vi "Crio9067_4chan.vi"() -> ()   [LabVIEW 2014]
uses:
  <vilib>/rvi/eio/common/nirviEmuClasses.ctl
  <vilib>/rvi/Emulation/niFpgaGetClockAttributes.vi
  <vilib>/rvi/Emulation/niFpgaSctlEmulationGetInTimedLoop.vi
  <vilib>/rvi/Emulation/niFpgaEmulationReportErrorSimple.vi
  <vilib>/rvi/Emulation/niFpgaProcessEmulError.vi
  <vilib>/rvi/eio/common/nirviEmuTemplateMethod_errors.vi
  <vilib>/rvi/Emulation/niFpgaCriticalErrorInLSC.vi
  <vilib>/rvi/interface/RandomDataEmulation/niFpgaRandomDataHandleErrors.vi
  <vilib>/eio/EIONode/EIONode.xnode
  <vilib>/eio/EIOGrowableMethodNode/genericMethod/EIOGrowableMethodNode.xnode
  <vilib>/rvi/eio/nirviEIOMethodImplementation/nirviEIOMethodImplementation.xnode
  <vilib>/rvi/eio/nirviErrorMerge/nirviErrorMerge.xnode
  <vilib>/rvi/DataTransferAndStorage/Container/XNode/niFpgaContainer.xnode
  <vilib>/rvi/interface/RandomDataEmulation/nirviRandomDataFpgaReadWriteTemplate.vi
panel:
  in  "User Fpga Led":bool
  out "Chassis Temperature":i16
  in  "System Reset":bool
  in  "Sample Period (uSec)":u32=2
  out "Timed Out":bool
  out "Overwrite":bool
  out "Sample Gated":bool
  in  "USER FPGA LED":bool
  in  "Boolean":bool
  out "Stopped":bool
  out "nChannels":i32=8
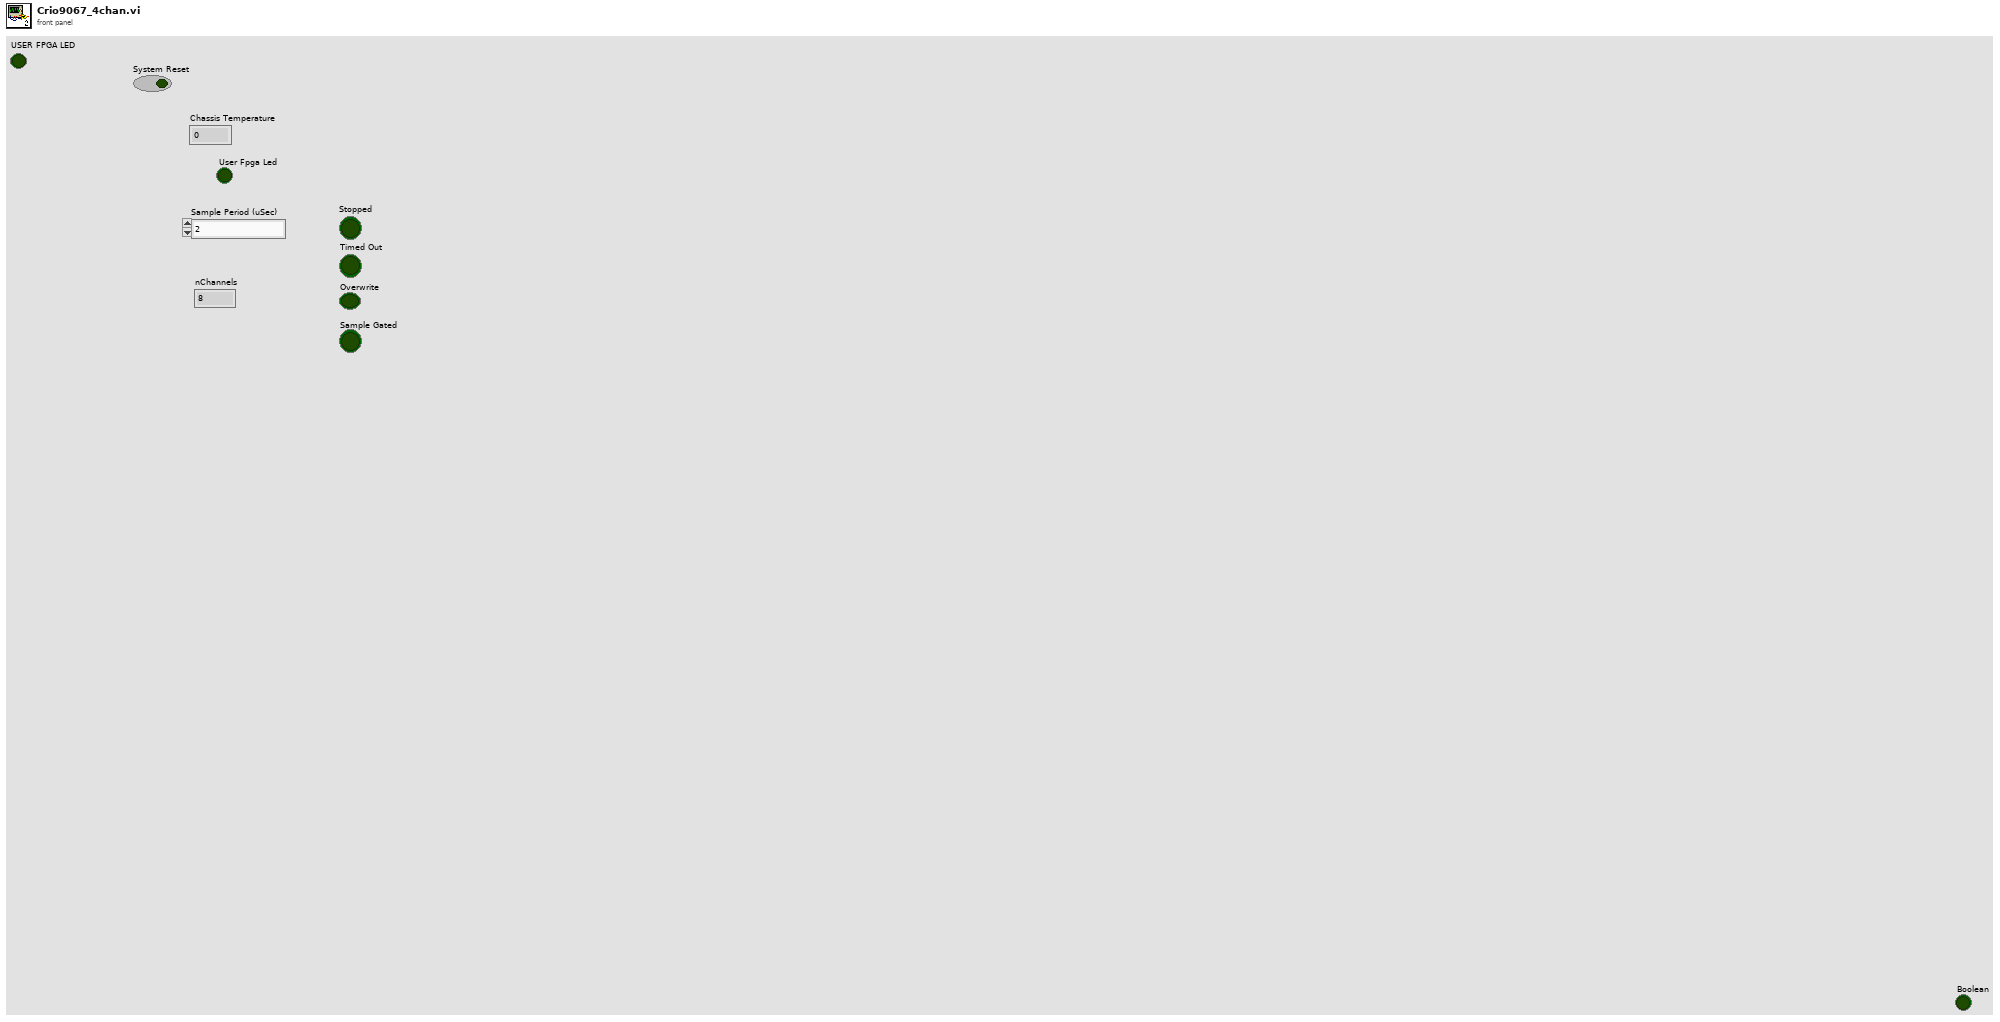
[diagram p1: front panel]
types:
  T1 = typedef "nirviEmuClasses.ctl" = enum16{"IO Read", "IO Write", "Method", "Property Read", "Property Write"}
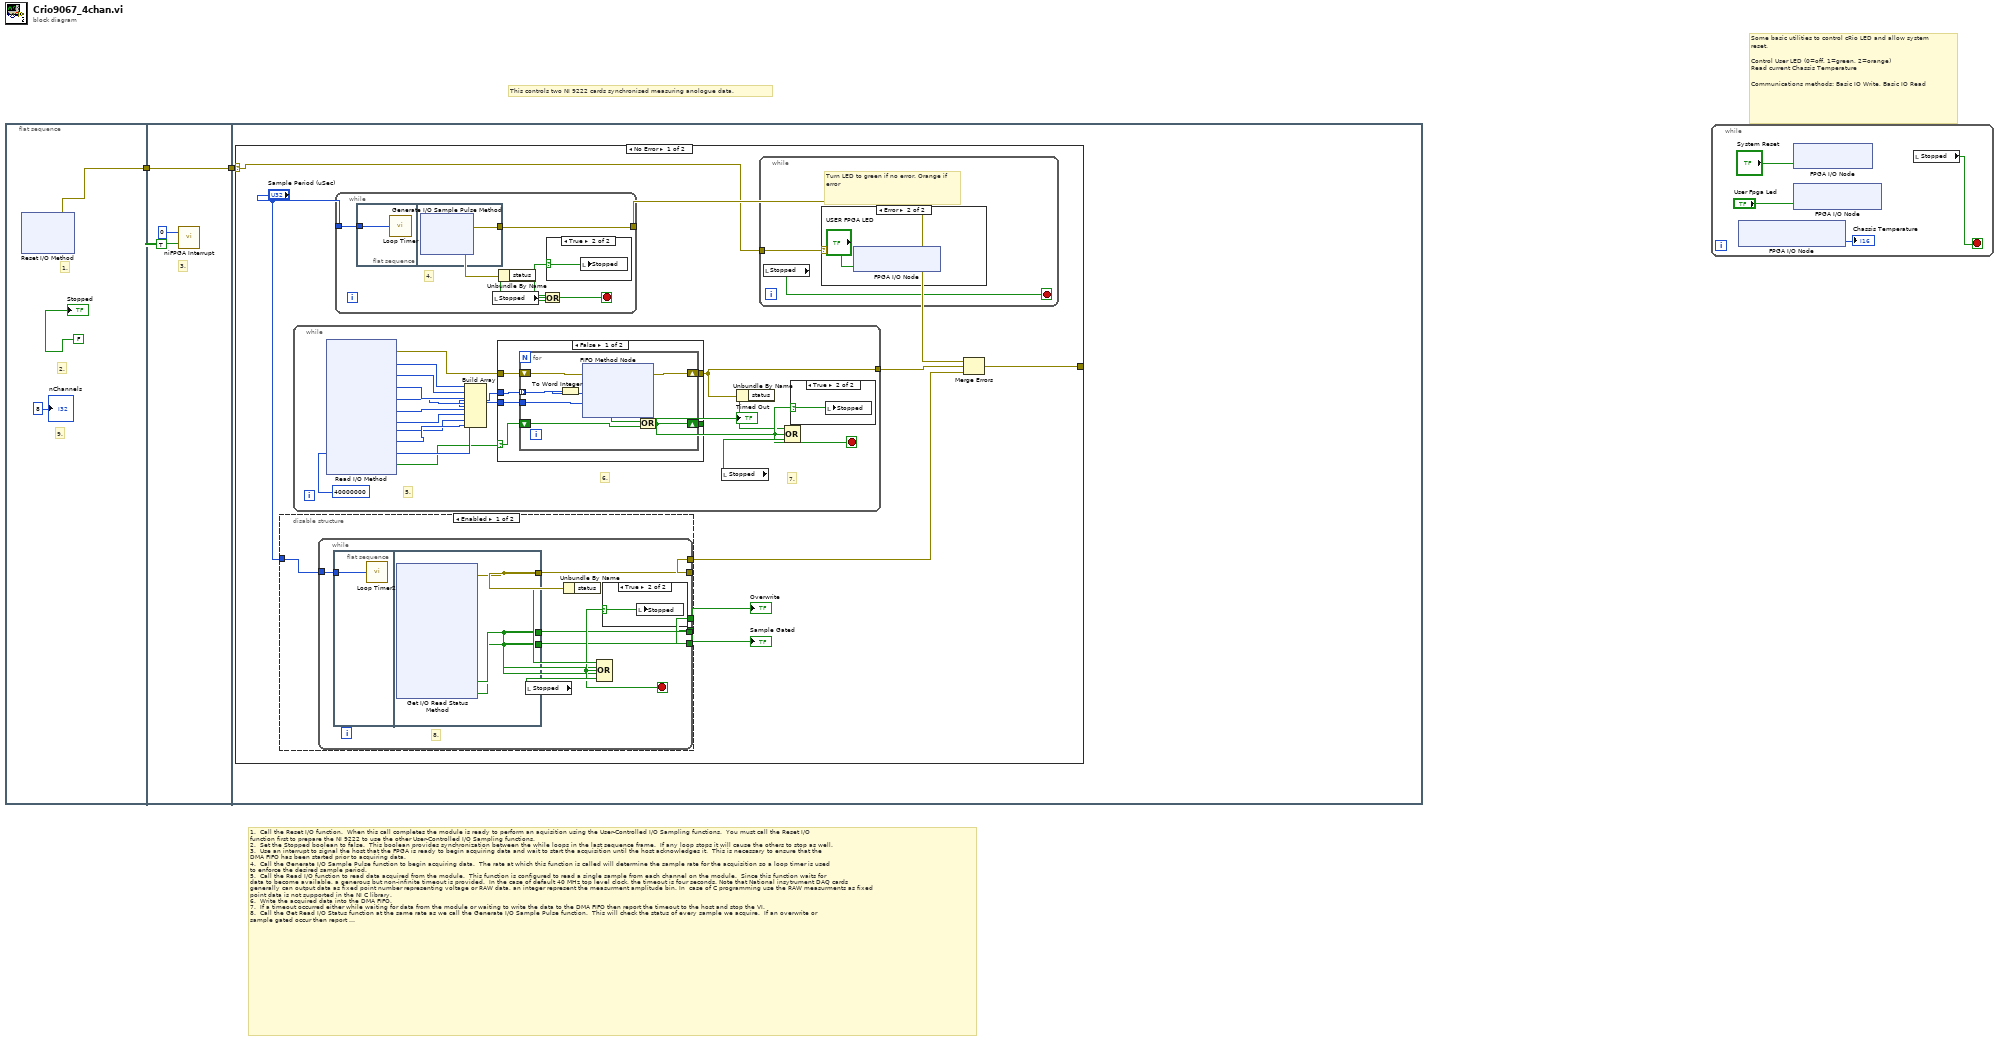
[diagram p0: block diagram]
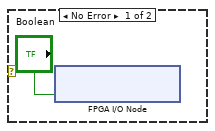
[diagram p2: hidden frame]
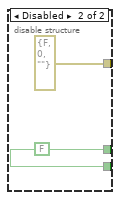
[diagram p4: hidden frame]
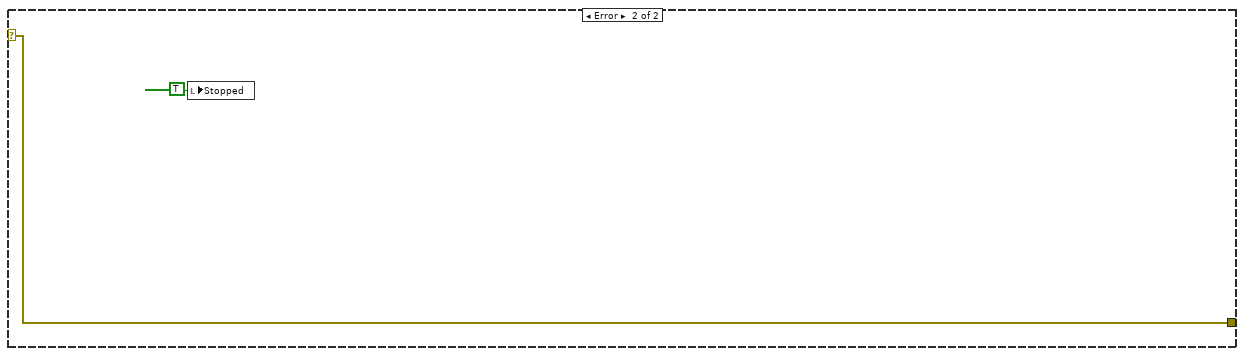
[diagram p8: hidden frame]
diagram:
  # "Some basic utilities to control cRio LED and allow system reset. \n\nControl User LED (0=off, 1=green, 2=orange)\nRead current Chassis Temperature\n\nCommunications methods: Basic IO Write, Basic IO Read"
  # "This controls two NI 9222 cards synchronised measuring anologue data."
  # "1.  Call the Reset I/O function.  When this call completes the module is ready to perform an aquisition using the User-Controlled I/O Sampling functions.  You must call the Reset I/O \nfunction first to prepare the NI 9222 to use the other User-Controlled I/O Sampling functions.\n2.  Set the Stopped boolean to false.  This boolean provides synchronization between the while loops in the last sequence frame.  If any loop stops it will cause the others to stop as well.\n3.  Use an interrupt to signal the host that the FPGA is ready to begin acquiring data and wait to start the acquisition until the host acknowledges it.  This is necessary to ensure that the \nDMA FIFO has been started prior to acquiring data.\n4.  Call the Generate I/O Sample Pulse function to begin acquiring data.  The rate at which this function is called will determine the sample rate for the acquisition so a loop timer is used\nto enforce the desired sample period.\n5.  Call the Read I/O function to read data acquired from the module.  This function is configured to read a single sample from each channel on the module.  Since this function waits for\ndata to become available, a generous but non-infinite timeout is provided.  In the case of default 40 MHz top level clock, the timeout is four seconds. Note that National insytrument DAQ cards \ngenerally can output data as fixed point number representing voltage or RAW data, an integer represent the measurment amplitude bin. In  case of C programming use the RAW measurments as fixed \npoint data is not supported in the NI C library. \n6.  Write the acquired data into the DMA FIFO.\n7.  If a timeout occurred either while waiting for data from the module or waiting to write the data to the DMA FIFO then report the timeout to the host and stop the VI.\n8.  Call the Get Read I/O Status function at the same rate as we call the Generate I/O Sample Pulse function.  This will check the status of every sample we acquire.  If an overwrite or \nsample gated occur then report the status to the host and stop the VI.  This loop is encased in a diagram disable struction to make it easily removable from the application.  Calling the \nGet Read I/O Status function is useful for development and debugging but not strictly necessary for deployment if there is no variable timing in the application.  In the above example, it\nis not possible to get a sample gated status unless the top loop's sample period is less than the minimum sample period supported by the module.  However, this application could \nproduce an overwrite status if the host VI cannot read from the DMA FIFO fast enough.\n9. I constant indicating the number of channels the FPGA is recording from. This is manually set."
  n1 = flat-sequence {
    tunnel: [w4] -> w2
    tunnel: w2 -> [w60]
    tunnel: [w60] -> w1
    tunnel: w1 -> [w63]
    frame #0 {
      # "9."
      # "2."
      # "1."
      n2 = xnode "Reset I/O Method"() -> ("error out"=w4:errorcluster)  [unwired: 3 in, 2 out]
      "Stopped" <- FALSE ("Stopped")
      "nChannels" <- 8
    }
    frame #1 {
      # "3."
      n3 = call <vilib>:"niFPGA Interrupt.vi"("Wait Until Cleared (F)"=TRUE ("Wait Until Cleared"), "IRQ Number (0)"=u8 0 ("IRQ Number")) -> ()  [unwired: 1 in]
    }
    frame #2 {
      n4 = case shown="No Error" w63 {
        selector: w63 -> [w64 w814]
        tunnel: [w68 w814] -> _
        frame No Error {
          n5 = disable-structure shown="Enabled" {
            disable-tunnel: [w79 errorcluster {"status"=FALSE, "code"=0, "source"=""} ("error out")] -> w69
            disable-tunnel: "Sample Period (uSec)" -> [w78 _]
            disable-tunnel: [w77 w392] -> w65
            disable-tunnel: [w76 w392] -> w66
            frame Enabled {
              n6 = while {
                tunnel: [w86] -> w79
                tunnel: w78 -> [w85]
                tunnel: [w81] -> w77
                tunnel: [w80] -> w76
                stop <- w82 stop-if-true
                # "8."
                n7 = flat-sequence {
                  tunnel: w85 -> [w88]
                  tunnel: [w91] -> w86
                  tunnel: [w90] -> w81
                  tunnel: [w89] -> w80
                  frame #0 {
                    n8 = call "Loop Timer2"("Count(uSec)"=w88) -> ()  [unwired: 1 out]
                  }
                  frame #1 {
                    n9 = xnode "Get I/O Read Status Method"() -> ("error out"=w91:errorcluster, "Overwrite"=w90:bool, "Sample Gated"=w89:bool)  [unwired: 9 in, 8 out]
                  }
                }
                n10 = local read "Stopped"() -> (w84:bool)
                n11 = Unbundle By Name(w86) -> ("status"=w83:bool)
                n12 = Compound Arithmetic op=OR(w83, w81, w80, w84) -> (w82:bool)
                n13 = case shown="True" w82 {
                  selector: w82 -> [_ w87]
                  frame False {
                  }
                  frame True {
                    n14 = local write "Stopped"(w87) -> ()
                  }
                }
              }
            }
            frame Disabled {
              w392 = FALSE ("Overwrite")
            }
          }
          "Overwrite" <- w65
          "Sample Gated" <- w66
          n15 = while {
            tunnel: [w408] -> w70
            stop <- w395 stop-if-true
            w409 = 40000000 ("Timeout")
            # "7."
            # "6."
            # "5."
            n16 = xnode "Read I/O Method"("Timeout"=w409) -> ("error out"=w407:errorcluster, "Mod1/AI0"=w397:i16, "Mod1/AI1"=w410:i16, "Mod1/AI2"=w403:i16, "Mod1/AI3"=w402:i16, "Mod2/AI0"=w401:i16, "Mod2/AI1"=w400:i16, "Mod2/AI2"=w398:i16, "Mod2/AI3"=w399:i16, "Timed Out"=w406:bool)  [unwired: 9 in, 8 out]
            n17 = Build Array(w397, w410, w403, w402, w401, w400, w398, w399) -> (w396:i16[])
            n18 = case shown="False" w406 {
              selector: w406 -> [w413 w426]
              tunnel: w409 -> [w417 _]
              tunnel: [w416 w427] -> w408
              tunnel: [w415 w426] -> w404
              tunnel: w407 -> [w414 w427]
              tunnel: w396 -> [w412 _]
              frame False {
                n19 = for {
                  tunnel: w412 -> [w418] mode=indexing
                  shift-right: [w424] -> w416
                  shift-left: w414 -> [w425]
                  tunnel: w417 -> [w423]
                  shift-right: [w421] -> w415
                  shift-left: w413 -> [w420]
                  n20 = To Word Integer(number=w418) -> (16bit integer=w419:i16)
                  n21 = xnode ("FIFO Method Node")("Element"=w419, "Timeout"=w423, "error in (no error)"=w425) -> ("Timed Out?"=w422:bool, "error out"=w424:errorcluster)  [unwired: 1 in, 1 out]
                  n22 = Or(x=w422, y=w420) -> (x .or. y?=w421:bool)
                }
              }
              frame True {
              }
            }
            "Timed Out" <- w404
            n23 = local read "Stopped"() -> (w405:bool)
            n24 = Unbundle By Name(w408) -> ("status"=w394:bool)
            n25 = Compound Arithmetic op=OR(w394, w404, w405) -> (w395:bool)
            n26 = case shown="True" w395 {
              selector: w395 -> [_ w411]
              frame False {
              }
              frame True {
                n27 = local write "Stopped"(w411) -> ()
              }
            }
          }
          n28 = while {
            tunnel: "Sample Period (uSec)" -> [w756]
            tunnel: [w753] -> w71
            stop <- w752 stop-if-true
            # "4."
            n29 = flat-sequence {
              tunnel: w756 -> [w758]
              tunnel: [w759] -> w753
              frame #0 {
                n30 = call "Loop Timer"("Count(uSec)"=w758) -> ()  [unwired: 1 out]
              }
              frame #1 {
                n31 = xnode "Generate I/O Sample Pulse Method"() -> ("error out"=w759:errorcluster)  [unwired: 3 in, 2 out]
              }
            }
            n32 = local read "Stopped"() -> (w755:bool)
            n33 = Unbundle By Name(w753) -> ("status"=w754:bool)
            n34 = Or(x=w754, y=w755) -> (x .or. y?=w752:bool)
            n35 = case shown="True" w752 {
              selector: w752 -> [_ w757]
              frame False {
              }
              frame True {
                n36 = local write "Stopped"(w757) -> ()
              }
            }
          }
          n37 = while {
            tunnel: w64 -> [w73]
            stop <- w72 stop-if-true
            # "Turn LED to green if no error. Orange if error"
            n38 = local read "Stopped"() -> (w72:bool)
            n39 = case shown="Error" w73 {
              frame No Error {
                n40 = xnode "FPGA I/O Node"("USER FPGA LED"="Boolean") -> ()  [unwired: 1 in, 1 out]
              }
              frame Error {
                n41 = xnode "FPGA I/O Node"("USER FPGA LED"="USER FPGA LED") -> ()  [unwired: 1 in, 1 out]
              }
            }
          }
          n42 = Merge Errors(w71, w70, w69) -> (w68:errorcluster)
        }
        frame Error {
          n43 = local write "Stopped"(TRUE ("Stopped")) -> ()
        }
      }
    }
  }
  n44 = while {
    stop <- w816 stop-if-true
    n45 = xnode "FPGA I/O Node"() -> ("Chassis Temperature"=→"Chassis Temperature":i16)  [unwired: 1 in, 1 out]
    n46 = xnode "FPGA I/O Node"("System Reset"="System Reset") -> ()  [unwired: 1 in, 1 out]
    n47 = xnode "FPGA I/O Node"("USER FPGA LED"="User Fpga Led") -> ()  [unwired: 1 in, 1 out]
    n48 = local read "Stopped"() -> (w816:bool)
  }
